vi "Write.EngineData.vi"(8 "error in":errorcluster, 11 "Write in":refnum<class "Write.lvclass">) -> (0 "error out":errorcluster, 3 "Write out":refnum<class "Write.lvclass">)   [LabVIEW 2027, in "Data Access Engine.lvlib" / "Write.lvclass"]
uses:
  Write.lvclass
  Write.lvclass/Write.ctl
  <vilib>/NI VeriStand/Custom Device API/Global Data Refs.vi
  <vilib>/NI VeriStand/Custom Device API/Custom Device API.lvlib
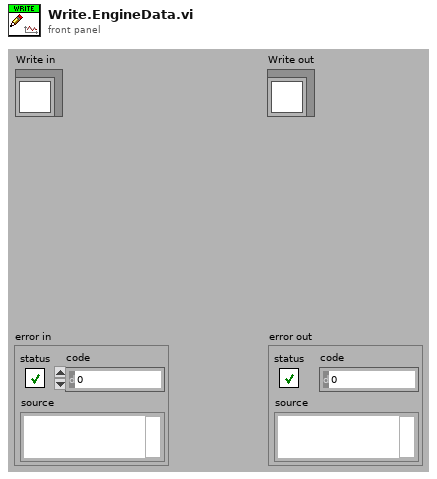
[diagram p1: front panel]
types:
  T1 = typedef "Custom Device API.lvlib/Block Data Reference.ctl" = cluster{"Data Reference":T2, "Offset":u64, "Length":u64}
  T2 = typedef "Custom Device API.lvlib/Data Reference.ctl" = i32
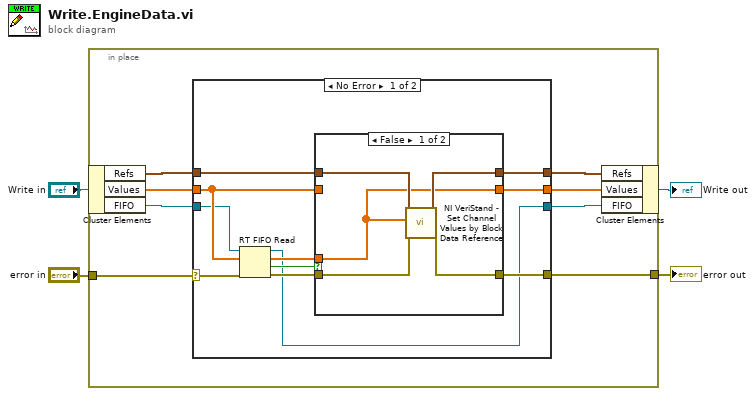
[diagram p0: block diagram]
diagram:
  n1 = in-place {
    in-place-border: [w12] -> w4
    in-place-border: "error in" -> [w7]
    n2 = in-place-cluster #1("Write in") -> ("Refs"=w11:T1[], "Values"=w10:dbl[], "FIFO"=w6:refnum<k33>)
    n3 = case shown="No Error" w7 {
      selector: w7 -> [w20 w35]
      tunnel: [w23 w35] -> w12
      tunnel: [w17 w34] -> w9
      tunnel: w11 -> [w16 w33]
      tunnel: w10 -> [w18 w34]
      tunnel: [w13 w33] -> w8
      tunnel: w6 -> [w15 w32]
      tunnel: [w14 w32] -> w5
      frame No Error {
        n4 = RT FIFO Read(0:w15, 1:w18, 3:w20) -> (8:w14:refnum<k33>, 9:w21:dbl[], 10:w19:bool, 11:w22:errorcluster)  [unwired: 1 in, 1 out]
        n5 = case shown="False" w19 {
          tunnel: w22 -> [w25 w31]
          tunnel: w21 -> [w26 _]
          tunnel: [w24 w31] -> w23
          tunnel: [w26 w30] -> w17
          tunnel: w16 -> [w28 w29]
          tunnel: w18 -> [_ w30]
          tunnel: [w27 w29] -> w13
          frame False {
            n6 = call <vilib>:"NI VeriStand - Set Channel Values by Block Data Reference.vi"("error in (no error)"=w25, "Values Array in"=w26, "Block Data Ref"=w28) -> ("error out"=w24:errorcluster, "Block Data Ref dup"=w27:T1[])  [unwired: 6 in, 1 out]
          }
          frame True {
          }
        }
      }
      frame Error {
      }
    }
    n7 = in-place-cluster #1("Refs"=w8, "Values"=w9, "FIFO"=w5) -> (→"Write out":refnum<class "Write.lvclass">)
  }
  "error out" <- w4
